vi "sub_read.vi"(4 "threshold":dbl=0.004, 6 "low":dbl=0.175, 7 "avg factor":dbl=0.8, 9 "high":dbl=0.215, 10 "x factor":dbl=0.2, 11 "Raw Signal":dynamicdata(waveform)) -> (1 "Digitized Sign":dynamicdata(waveform), 2 "Moving Avg":dynamicdata(waveform), 3 "Digital Signal":bool[](array[boolean]))   [LabVIEW 2015]
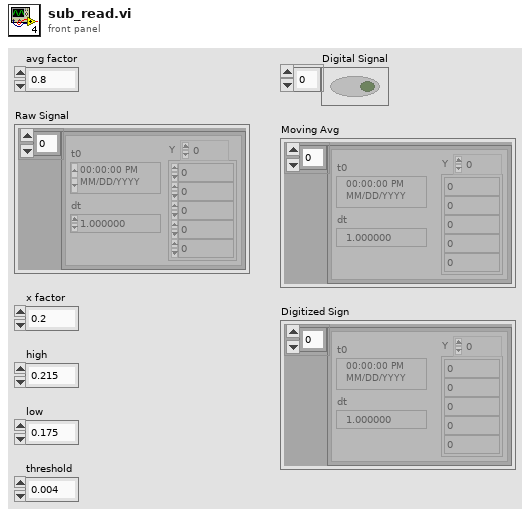
[diagram p1: front panel]
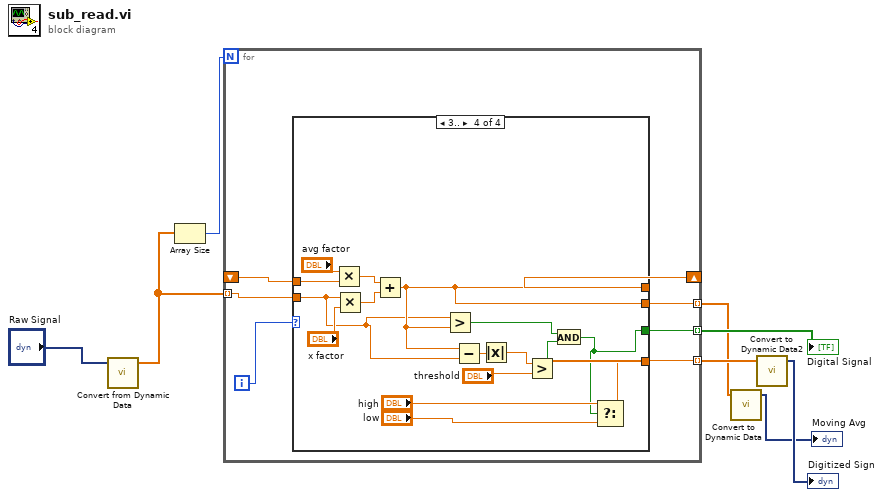
[diagram p0: block diagram]
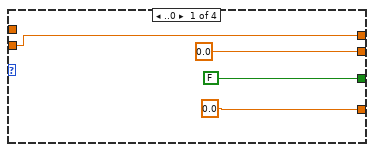
[diagram p2: hidden frame]
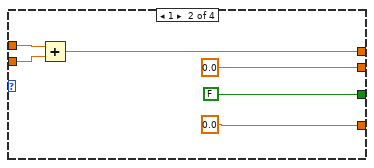
[diagram p3: hidden frame]
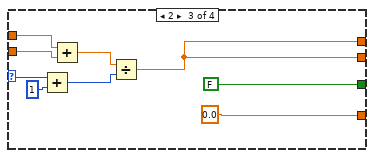
[diagram p4: hidden frame]
diagram:
  n1 = call "Convert from Dynamic Data"("Dynamic Data Type"="Raw Signal") -> ("Array"=w2:dbl[])  [unwired: 3 in]
  n2 = Array Size(array=w2) -> (size(s)=w1:i32)
  n3 = for {
    N: w1 -> [_]
    tunnel: w2 -> [w14] mode=indexing
    tunnel: [w13] -> w3 mode=indexing
    shift-right: [w11] -> _
    shift-left: _ -> [w12]
    tunnel: [w10] -> w6 mode=indexing
    tunnel: [w9] -> w7 mode=indexing
    i -> [w15]
    n4 = case shown="3.." w15 {
      selector: w15 -> [_ _ w31 _]
      tunnel: w14 -> [w18 w24 w30 w38]
      tunnel: [0.0 0.0 w28 w39] -> w13
      tunnel: w12 -> [_ w25 w29 w50]
      tunnel: [w18 w22 w28 w39] -> w11
      tunnel: [FALSE FALSE FALSE w35] -> w10
      tunnel: [0.0 ("low") 0.0 ("low") 0.0 ("low") w44] -> w9
      frame ..0 {
      }
      frame 1 {
        n5 = Add(x=w25, y=w24) -> (x+y=w22:dbl)
      }
      frame 2 {
        n6 = Add(x=w31, y=1) -> (x+y=w32:i32)
        n7 = Add(x=w29, y=w30) -> (x+y=w33:dbl)
        n8 = Divide(x=w33, y=w32) -> (x/y=w28:dbl)
      }
      frame 3.. {
        n9 = Multiply(x="avg factor", y=w50) -> (x*y=w47:dbl)
        n10 = Multiply(x=w38, y="x factor") -> (x*y=w46:dbl)
        n11 = Add(x=w47, y=w46) -> (x+y=w39:dbl)
        n12 = Greater?(x=w38, y=w39) -> (0:w36:bool)
        n13 = Subtract(x=w39, y=w38) -> (x-y=w42:dbl)
        n14 = Absolute Value(x=w42) -> (abs(x)=w41:dbl)
        n15 = Greater?(x=w41, y="threshold") -> (0:w37:bool)
        n16 = And(x=w36, y=w37) -> (x .and. y?=w35:bool)
        n17 = Select(t="high", s=w35, f="low") -> (s? t:f=w44:dbl)
      }
    }
  }
  "Digital Signal" <- w6
  n18 = call "Convert to Dynamic Data"("Array"=w3) -> ("Dynamic Data Type"=→"Moving Avg":dynamicdata)  [unwired: 3 in]
  n19 = call "Convert to Dynamic Data2"("Array"=w7) -> ("Dynamic Data Type"=→"Digitized Sign":dynamicdata)  [unwired: 3 in]
